vi "Send ConfigureMsg.vi"(8 "error in (no error)":errorcluster, 9 "filter":T1={"mode"=enum."Mirror", "levelMin"=enum."INFO", "levelMax"=enum."INFO", "tagPrefix"=""}, 10 "threshold":T3=enum."INFO", 11 "Enqueuer in":refnum<class "Message Enqueuer.lvclass">) -> (0 "error out":errorcluster, 3 "Enqueuer out":refnum<class "Message Enqueuer.lvclass">)   [LabVIEW 2026, in "Lumberjack.lvlib" / "ConfigureMsg.lvclass"]
uses:
  ConfigureMsg.lvclass
  <vilib>/ActorFramework/Message Enqueuer/Message Enqueuer.lvclass
  TypeDefs/Severity.ctl
  TypeDefs/Filter.ctl
  TypeDefs/FilterMode.ctl
  ConfigureMsg.lvclass/ConfigureMsg.ctl
  <vilib>/ActorFramework/Message Enqueuer/Message Enqueuer.lvclass/Message Enqueuer.ctl
  <vilib>/ActorFramework/Message Priority Queue/Priority Enqueue.vi
  Lumberjack.lvlib
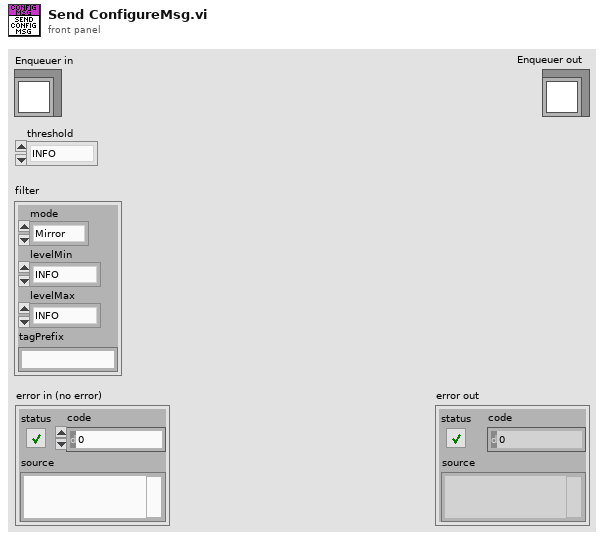
[diagram p1: front panel]
types:
  T1 = typedef "Lumberjack.lvlib/Filter.ctl" = cluster{"mode":T2, "levelMin":T3, "levelMax":T3, "tagPrefix":string}
  T2 = typedef "Lumberjack.lvlib/FilterMode.ctl" = enum16{"Mirror", "Routed"}
  T3 = typedef "Lumberjack.lvlib/Severity.ctl" = enum16{"OFF", "FATAL", "ERROR", "WARN", "INFO", "DEBUG", "TRACE", "ALL"}
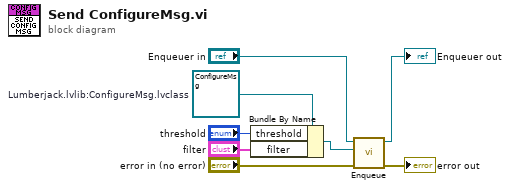
[diagram p0: block diagram]
diagram:
  w5 = refnum<class "ConfigureMsg.lvclass"> refnum  # Lumberjack.lvlib:ConfigureMsg.lvclass
  n1 = Bundle By Name(cluster=w5, "threshold"="threshold", "filter"="filter") -> (w2:refnum<class "ConfigureMsg.lvclass">)
  n2 = call <vilib>:"Enqueue.vi"("error in (no error)"="error in (no error)", "Message"=w2, "Message Enqueuer in"="Enqueuer in") -> ("error out"=→"error out":errorcluster, "Message Enqueuer out"=→"Enqueuer out":refnum<class "Message Enqueuer.lvclass">)  [unwired: 7 in]
